vi "HFRR ADV v02.vi"() -> ()   [LabVIEW 2023] (continued)
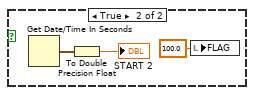
[diagram p4: hidden frame]
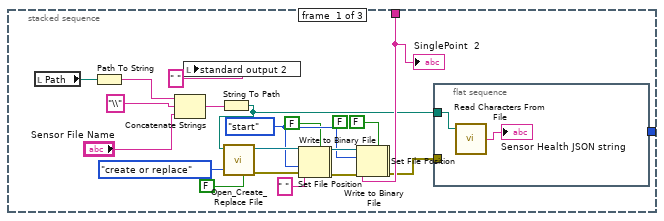
[diagram p9: hidden frame]
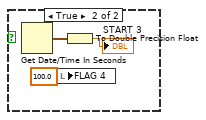
[diagram p13: hidden frame]
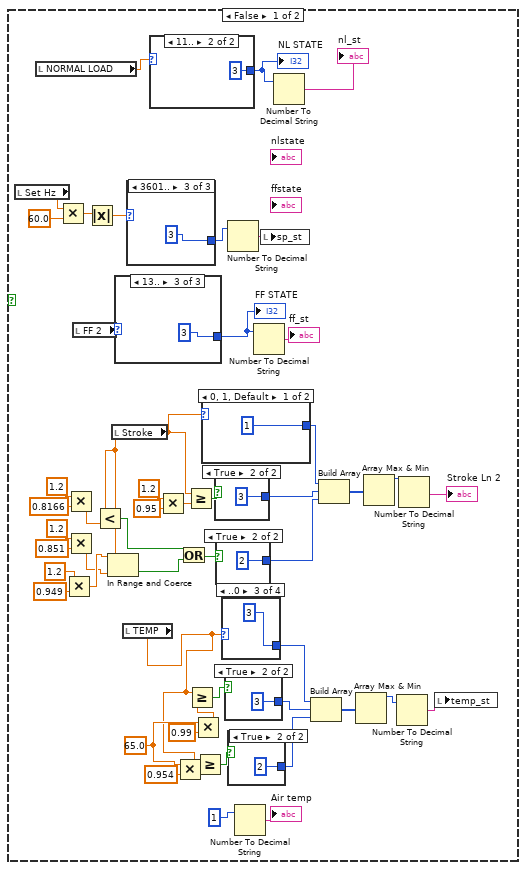
[diagram p15: hidden frame]
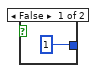
[diagram p16: hidden frame]
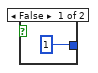
[diagram p17: hidden frame]
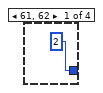
[diagram p18: hidden frame]
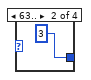
[diagram p19: hidden frame]
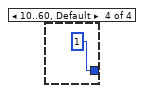
[diagram p20: hidden frame]
                n2644 = Multiply(x=1.2 ("y"), y=0.8166) -> (x*y=w3925:dbl)
                n2645 = Multiply(x=1.2 ("y"), y=0.851) -> (x*y=w3920:dbl)
                n2646 = local read "FF 2"() -> (w3944:dbl)
                n2647 = Absolute Value(x=w3952) -> (abs(x)=w3950:dbl)
                n2648 = local read "Stroke"() -> (w3919:dbl)
                n2649 = Less?(x=w3919, y=w3925) -> (x < y?=w3922:bool)
                n2650 = In Range and Coerce(upper limit=w3921, x=w3919, lower limit=w3920) -> (In Range?=w3923:bool)  [unwired: 1 out]
                n2651 = case shown="13.." w3944 {
                  tunnel: [1 2 3] -> w3942
                  frame 0..10, Default {
                    # "Normal"
                  }
                  frame 11, 12 {
                  }
                  frame 13.. {
                  }
                }
                "FF STATE" <- w3942
                n2652 = local read "TEMP"() -> (w3905:dbl)
                n2653 = case shown="3601.." w3950 {
                  tunnel: [1 2 3] -> w3948
                  frame 0..3000, Default {
                    # "Normal"
                  }
                  frame 3001..3600 {
                  }
                  frame 3601.. {
                  }
                }
                n2654 = case shown="11.." w3946 {
                  tunnel: [1 3] -> w3947
                  frame 1..10, Default {
                  }
                  frame 11.. {
                  }
                }
                "NL STATE" <- w3947
                n2655 = Multiply(x=1.2 ("y"), y=0.95) -> (x*y=w3935:dbl)
                n2656 = Multiply(x=w3917, y=0.954) -> (x*y=w3909:dbl)
                n2657 = Or(x=w3922, y=w3923) -> (x .or. y?=w3924:bool)
                n2658 = Greater Or Equal?(x=w3919, y=w3935) -> (x >= y?=w3932:bool)
                n2659 = Multiply(x=w3917, y=0.99) -> (x*y=w3906:dbl)
                n2660 = Greater Or Equal?(x=w3905, y=w3906) -> (x >= y?=w3911:bool)
                n2661 = Greater Or Equal?(x=w3905, y=w3909) -> (x >= y?=w3908:bool)
                n2662 = case shown="0, 1, Default" w3919 {
                  tunnel: [1 3] -> w3936
                  frame 0, 1, Default {
                  }
                  frame 2.. {
                  }
                }
                n2663 = case shown="True" w3932 {
                  tunnel: [1 3] -> w3937
                  frame False {
                  }
                  frame True {
                  }
                }
                n2664 = case shown="True" w3924 {
                  tunnel: [1 2] -> w3938
                  frame False {
                  }
                  frame True {
                  }
                }
                n2665 = case shown="..0" w3905 {
                  tunnel: [2 3 3 1] -> w3912
                  frame 61, 62 {
                  }
                  frame 63.. {
                  }
                  frame ..0 {
                  }
                  frame 10..60, Default {
                  }
                }
                n2666 = case shown="True" w3911 {
                  tunnel: [1 3] -> w3913
                  frame False {
                  }
                  frame True {
                  }
                }
                n2667 = Number To Decimal String(number=w3948) -> (decimal integer string=w3949:string)  [unwired: 1 in]
                n2668 = case shown="True" w3908 {
                  tunnel: [1 2] -> w3914
                  frame False {
                  }
                  frame True {
                  }
                }
                n2669 = Number To Decimal String(number=1) -> (decimal integer string=→"Air temp":string)  [unwired: 1 in]
                n2670 = Number To Decimal String(number=w3942) -> (decimal integer string=→"ff_st":string)  [unwired: 1 in]
                n2671 = local write "sp_st"(w3949) -> ()
                n2672 = Number To Decimal String(number=w3947) -> (decimal integer string=→"nl_st":string)  [unwired: 1 in]
                n2673 = Build Array(w3912, w3913, w3914) -> (w3915:i32[])
                n2674 = Build Array(w3936, w3937, w3938) -> (w3939:i32[])
                n2675 = Array Max & Min(array=w3915) -> (max value=w3916:i32)  [unwired: 3 out]
                n2676 = Array Max & Min(array=w3939) -> (max value=w3940:i32)  [unwired: 3 out]
                n2677 = Number To Decimal String(number=w3916) -> (decimal integer string=w3904:string)  [unwired: 1 in]
                n2678 = Number To Decimal String(number=w3940) -> (decimal integer string=→"Stroke Ln 2":string)  [unwired: 1 in]
                n2679 = local write "temp_st"(w3904) -> ()
              }
              frame True {
                w4002 = 65.0 ("y")
                # "Healthy -1\nWarning -2\nError -3"
                n2680 = local read "TEMP"() -> (w4013:dbl)
                n2681 = local read "NORMAL LOAD"() -> (w4017:dbl)
                n2682 = local read "Set Hz"() -> (w4015:dbl)
                n2683 = Multiply(x=1.2 ("y"), y=0.949) -> (x*y=w3997:dbl)
                n2684 = Multiply(x=1.2 ("y"), y=0.8166) -> (x*y=w3993:dbl)
                n2685 = Multiply(x=1.2 ("y"), y=0.851) -> (x*y=w3998:dbl)
                n2686 = Multiply(x=w4002, y=0.954) -> (x*y=w4009:dbl)
                n2687 = Multiply(x=w4002, y=0.99) -> (x*y=w4012:dbl)
                n2688 = Greater Or Equal?(x=w4013, y=w4012) -> (x >= y?=w4007:bool)
                n2689 = Multiply(x=w4015, y=60.0) -> (x*y=w4021:dbl)
                n2690 = Greater Or Equal?(x=w4013, y=w4009) -> (x >= y?=w4010:bool)
                n2691 = local read "FF 2"() -> (w4016:dbl)
                n2692 = local read "Stroke"() -> (w3999:dbl)
                n2693 = Less?(x=w3999, y=w3993) -> (x < y?=w3996:bool)
                n2694 = In Range and Coerce(upper limit=w3997, x=w3999, lower limit=w3998) -> (In Range?=w3995:bool)  [unwired: 1 out]
                n2695 = Absolute Value(x=w4021) -> (abs(x)=w4019:dbl)
                n2696 = case shown="63.." w4013 {
                  tunnel: [2 3 3 1] -> w4006
                  frame 61, 62 {
                  }
                  frame 63.. {
                  }
                  frame ..0 {
                  }
                  frame 10..60, Default {
                  }
                }
                n2697 = case shown="True" w4007 {
                  tunnel: [1 3] -> w4005
                  frame False {
                  }
                  frame True {
                  }
                }
                n2698 = case shown="True" w4010 {
                  tunnel: [1 2] -> w4004
                  frame False {
                  }
                  frame True {
                  }
                }
                n2699 = Multiply(x=1.2 ("y"), y=0.95) -> (x*y=w3983:dbl)
                n2700 = case shown="1..10, Default" w4017 {
                  tunnel: [1 3] -> w4024
                  frame 1..10, Default {
                  }
                  frame 11.. {
                  }
                }
                n2701 = case shown="0..10, Default" w4016 {
                  tunnel: [1 2 3] -> w4023
                  frame 0..10, Default {
                  }
                  frame 11, 12 {
                  }
                  frame 13.. {
                  }
                }
                n2702 = case shown="3601.." w4019 {
                  tunnel: [1 2 3] -> w4018
                  frame 0..3000, Default {
                    # "Normal"
                  }
                  frame 3001..3600 {
                  }
                  frame 3601.. {
                  }
                }
                n2703 = Or(x=w3996, y=w3995) -> (x .or. y?=w3994:bool)
                n2704 = Greater Or Equal?(x=w3999, y=w3983) -> (x >= y?=w3986:bool)
                n2705 = case shown="0, 1, Default" w3999 {
                  tunnel: [1 3] -> w3982
                  frame 0, 1, Default {
                  }
                  frame 2.. {
                  }
                }
                n2706 = case shown="True" w3986 {
                  tunnel: [1 3] -> w3981
                  frame False {
                  }
                  frame True {
                  }
                }
                n2707 = case shown="True" w3994 {
                  tunnel: [1 2] -> w3980
                  frame False {
                  }
                  frame True {
                  }
                }
                n2708 = Build Array(w4006, w4005, w4004) -> (w4003:i32[])
                n2709 = Number To Decimal String(number=w4018) -> (decimal integer string=→"sp_st":string)  [unwired: 1 in]
                n2710 = Array Max & Min(array=w4003) -> (max value=w4000:i32)  [unwired: 3 out]
                "TEMP STATE" <- w4000
                n2711 = Number To Decimal String(number=w4024) -> (decimal integer string=w4027:string)  [unwired: 1 in]
                n2712 = Number To Decimal String(number=w4023) -> (decimal integer string=w4025:string)  [unwired: 1 in]
                n2713 = Number To Decimal String(number=w4000) -> (decimal integer string=→"temp_st":string)  [unwired: 1 in]
                n2714 = Build Array(w3982, w3981, w3980) -> (w3979:i32[])
                n2715 = local write "nl_st"(w4027) -> ()
                n2716 = local write "ff_st"(w4025) -> ()
                n2717 = Number To Decimal String(number=1) -> (decimal integer string=w4022:string)  [unwired: 1 in]
                n2718 = Array Max & Min(array=w3979) -> (max value=w3978:i32)  [unwired: 3 out]
                n2719 = local write "Air temp"(w4022) -> ()
                n2720 = Number To Decimal String(number=w3978) -> (decimal integer string=w3977:string)  [unwired: 1 in]
                n2721 = local write "Stroke Ln 2"(w3977) -> ()
              }
            }
            n2722 = local read "Stroke Ln 2"() -> (w3889:string)
            n2723 = local read "nl_st"() -> (w3895:string)
            n2724 = local read "ff_st"() -> (w3892:string)
            n2725 = local read "sp_st"() -> (w3893:string)
            n2726 = local read "temp_st"() -> (w3894:string)
            n2727 = local read "Air temp"() -> (w3888:string)
            n2728 = Replace Array Subset(array="in", new element #1=w3895, index #1=1 ("index"), new element #2=w3892, index #2=2 ("index"), new element #3=w3894, index #3=3 ("index"), new element #4=w3893, index #4=4 ("index"), new element #5=w3889, index #5=5 ("index"), new element #6=w3888, index #6=6 ("index"), new element #7="Sensor State" ("new element/subarray"), index #7=0 ("index")) -> (→"out":string[])
          }
        }
        n2729 = Wait (ms)(milliseconds to wait=u32 10) -> ()  [unwired: 1 out]
        n2730 = local read "EXIT"() -> (w3884:bool)
      }
      n2731 = while {
        stop <- w3858 stop-if-true
        n2732 = local read "run replace"() -> (w3860:bool)
        n2733 = Wait (ms)(milliseconds to wait=u32 100) -> ()  [unwired: 1 out]
        n2734 = Equal?(x="FLAG 2", y=0.0) -> (x = y?=w3861:bool)
        n2735 = case shown="True" w3861 {
          frame False {
          }
          frame True {
            n2736 = local write "FLAG 2"(100.0 ("FLAG 2")) -> ()
            n2737 = call <vilib>:"Read Characters From File.vi"("file path (dialog if empty)"=path "C:/LAB-IQ-NXT/WO 2449 TT.sig", "convert eol? (no:F)"=FALSE ("append to file? (new file:F)")) -> ("character string"=w3864:string)  [unwired: 4 in, 3 out]
            n2738 = call <vilib>:"Read Characters From File.vi"("file path (dialog if empty)"=path "C:/LAB-IQ-NXT/WO 2449 TRH.sig", "convert eol? (no:F)"=FALSE ("append to file? (new file:F)")) -> ("character string"=w3865:string)  [unwired: 4 in, 3 out]
            n2739 = Decimal String To Number(string=w3864) -> (number=w3866:i32)  [unwired: 2 in, 1 out]
            n2740 = local write "Total No. of Tests"(w3866) -> ()
            n2741 = Decimal String To Number(string=w3865) -> (number=w3869:i32)  [unwired: 2 in, 1 out]
            n2742 = local write "SEN.RUN HRS"(w3869) -> ()
          }
        }
        n2743 = case shown="True" w3860 {
          frame False {
          }
          frame True {
            n2744 = Equal?(x="FLAG 4", y=0.0) -> (x = y?=w3873:bool)
            n2745 = case shown="False" w3873 {
              frame False {
                n2746 = Get Date/Time In Seconds() -> (seconds since 1Jan1904=w3879:timestamp)
                n2747 = local read "START 3"() -> (w3877:dbl)
                n2748 = To Double Precision Float(number=w3879) -> (double precision float=w3878:dbl)
                n2749 = Subtract(x=w3878, y=w3877) -> (x-y=→"SENSOR TIME":dbl)
              }
              frame True {
                n2750 = Get Date/Time In Seconds() -> (seconds since 1Jan1904=w3881:timestamp)
                n2751 = local write "FLAG 4"(100.0 ("FLAG")) -> ()
                n2752 = To Double Precision Float(number=w3881) -> (double precision float=→"START 3":dbl)
              }
            }
          }
        }
        n2753 = local read "EXIT"() -> (w3858:bool)
      }
      n2754 = while {
        shift-right: [w3656] -> _
        shift-left: _ -> [w3657]
        tunnel: [w3651] -> _
        i -> [w3651]
        stop <- w3650 stop-if-true
        n2755 = Wait (ms)(milliseconds to wait=u32 50 ("Refresh Rate (ms)")) -> ()  [unwired: 1 out]
        n2756 = local read "Json End Flg"() -> (w3652:bool)
        n2757 = Not(x="Upld AR 2") -> ()  [unwired: 1 out]
        n2758 = local read "Upld AR 2"() -> (w3653:bool)
        n2759 = call "Elapsed Time9"("Time Target (s)"="Sen.Upload Rate (s)", "Reset"=FALSE, "Auto Reset"=TRUE) -> ("Time has Elapsed"=w3663:bool)  [unwired: 9 in, 7 out]
        n2760 = Or(x=w3663, y=w3652) -> (x .or. y?=w3659:bool)
        n2761 = case shown="True" w3659 {
          frame False {
          }
          frame True {
            w3757 = "\"SensorName\":\"" ("string")
            w3727 = " \"},{"
            w3752 = "\",\"SensorState\":\""
            w3754 = "\",\"SensorModelNumber\":\"" ("string")
            w3753 = "\",\"SensorRuntimeHours\":\"" ("string")
            n2762 = local read "model num"() -> (w3751:string[])
            n2763 = local read "Sensor name"() -> (w3770:string[])
            n2764 = local read "run"() -> (w3741:string[])
            n2765 = local read "SENSOR TIME"() -> (w3696:dbl)
            n2766 = local read "out"() -> (w3689:string[])
            n2767 = local read "Total No. of Tests"() -> (w3694:dbl)
            n2768 = Select(t=60.0, s="Run test 3", f=3600.0) -> (s? t:f=w3705:dbl)
            n2769 = Index Array(array=w3751, index #1=1 ("index")) -> (element #1=w3750:string, element #2=w3749:string, element #3=w3748:string, element #4=w3747:string, element #5=w3746:string, element #6=w3745:string)  [unwired: 5 in]
            n2770 = Index Array(array=w3741, index #1=1 ("index")) -> (element #1=w3740:string, element #2=w3739:string, element #3=w3738:string, element #4=w3737:string, element #5=w3736:string, element #6=w3735:string)  [unwired: 5 in]
            n2771 = Index Array(array=w3770, index #1=1 ("index")) -> (element #1=w3769:string, element #2=w3768:string, element #3=w3767:string, element #4=w3766:string, element #5=w3756:string, element #6=w3755:string)  [unwired: 5 in]
            n2772 = Index Array(array=w3689, index #1=1 ("index")) -> (element #1=w3722:string, element #2=w3721:string, element #3=w3720:string, element #4=w3719:string, element #5=w3718:string, element #6=w3717:string)  [unwired: 5 in]
            n2773 = local read "SEN.RUN HRS"() -> (w3692:dbl)
            n2774 = Divide(x=w3696, y=w3705) -> (x/y=w3704:dbl)
            n2775 = Increment(x=w3704) -> (x+1=w3699:dbl)
            n2776 = Number To Decimal String(number=w3699) -> (decimal integer string=→"run hrs":string)  [unwired: 1 in]
            n2777 = Divide(x=w3692, y=3600.0 ("f")) -> (x/y=w3687:dbl)
            n2778 = Round To Nearest(number=w3687) -> (nearest integer value=w3685:dbl)
            n2779 = Number To Decimal String(number=w3685) -> (decimal integer string=w3686:string)  [unwired: 1 in]
            n2780 = Number To Decimal String(number=w3694) -> (decimal integer string=w3695:string)  [unwired: 1 in]
            n2781 = local read "Model No"() -> (w3700:string)
            n2782 = local read "UUID"() -> (w3796:string)
            n2783 = local read "Serial No"() -> (w3800:string)
            n2784 = local read "Secret Key"() -> (w3801:string)
            n2785 = Concatenate Strings("\",\"MachineSerialNumber\":\"" ("string"), w3800) -> (w3804:string)
            n2786 = Concatenate Strings("\",\"ModelNumber\":\"" ("string"), w3700) -> (w3701:string)
            n2787 = Concatenate Strings("\",\"MachineRuntimeHours\":\"" ("string"), w3686) -> (w3805:string)
            n2788 = Concatenate Strings("\",\"MachineRuntimeCycles\":\"", w3695) -> (w3798:string)
            n2789 = Concatenate Strings(w3754, w3750) -> (w3784:string)
            n2790 = Concatenate Strings(w3753, w3740) -> (w3785:string)
            n2791 = Concatenate Strings(w3752, w3722) -> (w3783:string)
            n2792 = Concatenate Strings(w3804, w3701, w3805, w3798) -> (w3807:string)
            n2793 = Concatenate Strings(w3754, w3749) -> (w3781:string)
            n2794 = Concatenate Strings(w3753, w3739) -> (w3780:string)
            n2795 = Concatenate Strings(w3752, w3721) -> (w3782:string)
            n2796 = Concatenate Strings(w3754, w3748) -> (w3776:string)
            n2797 = Concatenate Strings(w3753, w3738) -> (w3777:string)
            n2798 = Concatenate Strings(w3752, w3720) -> (w3775:string)
            n2799 = Concatenate Strings(w3754, w3747) -> (w3773:string)
            n2800 = Concatenate Strings(w3753, w3737) -> (w3772:string)
            n2801 = Concatenate Strings(w3752, w3719) -> (w3774:string)
            n2802 = Concatenate Strings(w3784, w3785, w3783) -> (w3786:string)
            n2803 = Concatenate Strings(w3754, w3746) -> (w3763:string)
            n2804 = Concatenate Strings(w3753, w3736) -> (w3764:string)
            n2805 = Concatenate Strings(w3754, w3745) -> (w3760:string)
            n2806 = Concatenate Strings(w3753, w3735) -> (w3759:string)
            n2807 = Concatenate Strings(w3752, w3718) -> (w3762:string)
            n2808 = Concatenate Strings(w3752, w3717) -> (w3761:string)
            n2809 = Concatenate Strings("{\"SecretKey\":\"", w3801, w3807, "\",\"UUID\" : \"", w3796, "\",\"SensorInformation\":", "[{" ("string")) -> (w3734:string)
            n2810 = Concatenate Strings(w3781, w3780, w3782) -> (w3779:string)
            n2811 = Concatenate Strings(w3776, w3777, w3775) -> (w3778:string)
            n2812 = Concatenate Strings(w3773, w3772, w3774) -> (w3771:string)
            n2813 = Concatenate Strings(w3763, w3764, w3762) -> (w3765:string)
            n2814 = Concatenate Strings(w3760, w3759, w3761) -> (w3758:string)
            n2815 = Concatenate Strings(w3757, w3769, w3786, w3727) -> (w3733:string)
            n2816 = Concatenate Strings(w3757, w3768, w3779, w3727) -> (w3732:string)
            n2817 = Concatenate Strings(w3757, w3767, w3778, w3727) -> (w3731:string)
            n2818 = Concatenate Strings(w3757, w3766, w3771, w3727) -> (w3730:string)
            n2819 = Concatenate Strings(w3757, w3756, w3765, w3727) -> (w3729:string)
            n2820 = Concatenate Strings(w3757, w3755, w3758, "\"}" ("string")) -> (w3728:string)
            n2821 = Concatenate Strings(w3734, w3733, w3732, w3731, w3730, w3729, w3728, "]}" ("string")) -> (w3725:string)
            n2822 = local read "SEN.RUN HRS"() -> (w3691:dbl)
            n2823 = case shown="True" "Case Constant\n(See Context Help) 3" {
              frame False {
              }
              frame True {
                n2824 = local read "state"() -> (w3811:string[])
                n2825 = Delete From Array(array=w3811, index=0) -> (array with subset deleted=w3809:string[])  [unwired: 1 in, 1 out]
                n2826 = for {
                  N: 6 -> [_]
                  tunnel: w3809 -> [w3822] mode=indexing
                  tunnel: [w3821] -> w3808 mode=indexing
                  n2827 = Equal?(x=w3822, y="Warning") -> (x = y?=w3818:bool)
                  n2828 = Equal?(x=w3822, y="Healthy") -> (x = y?=w3815:bool)
                  n2829 = Select(t="2" ("y"), s=w3818, f="3" ("y")) -> (s? t:f=w3813:string)
                  n2830 = Select(t="1" ("y"), s=w3815, f=w3813) -> (s? t:f=w3821:string)
                }
                "state1" <- w3808
              }
            }
            n2831 = stacked-sequence {
              tunnel: w3725 -> [w3833 _ _]
              tunnel: [_ _ w3849] -> _
              frame #0 {
                (unwired) FALSE ("convert eol (F)")
                w3835 = enum16{"start", "end", "current"}."start" ("pos mode (0:2)")
                n2832 = local read "Path"() -> (w3829:path)
                n2833 = Path To String(path=w3829) -> (string=w3841:string)
                n2834 = Concatenate Strings(w3841, "\\", "Sensor File Name") -> (w3842:string)
                n2835 = local write "standard output 2"(" ") -> ()
                n2836 = String To Path(string=w3842) -> (path=w3832:path)
                n2837 = call <vilib>:"Open_Create_Replace File.vi"("advisory dialog? (display:T)"=FALSE, "function (open:0)"=T16."create or replace", "file path"=w3832) -> ("error out"=w3845:errorcluster, "refnum"=w3844:refnum<file>)  [unwired: 5 in, 2 out]
                n2838 = Set File Position(refnum=w3844, from (0:start)=w3835, error in=w3845) -> (refnum out=w3825:refnum<file>, error out=w3824:errorcluster)  [unwired: 1 in]
                n2839 = Write to Binary File(file (use dialog)=w3825, data=" ", error in=w3824, 5:FALSE ("prepend array or string size? (T)")) -> (refnum out=w3836:refnum<file>, error out=w3837:errorcluster)  [unwired: 2 in, 1 out]
                n2840 = Set File Position(offset (in bytes) (0)=w3835, refnum=w3836, error in=w3837) -> (refnum out=w3828:refnum<file>, error out=w3827:errorcluster)  [unwired: 1 in]
                n2841 = Write to Binary File(file (use dialog)=w3828, data=w3833, error in=w3827, 5:FALSE ("prepend array or string size? (T)")) -> (error out=w3831:errorcluster)  [unwired: 2 in, 2 out]
                n2842 = flat-sequence {
                  tunnel: w3832 -> [w3847]
                  tunnel: w3831 -> [_]
                  frame #0 {
                    n2843 = call <vilib>:"Read Characters From File.vi"("file path (dialog if empty)"=w3847) -> ("character string"=→"Sensor Health JSON string":string)  [unwired: 5 in, 3 out]
                  }
                }
                "SinglePoint  2" <- w3833
              }
              frame #1 {
              }
              frame #2 {
                (unwired) "\"Stored\": true" ("string")
                n2844 = call <vilib>:"System Exec.vi"("run minimized? (F)"=TRUE, "wait until completion? (T)"=TRUE, "working directory"=path "C:/LAB-IQ-NXT", "command line"="C:\\LAB-IQ-NXT\\JPostH.bat") -> ("standard error"=→"Respose From Server 2":string, "standard output"=w3852:string)  [unwired: 4 in, 2 out]
                "standard output 2" <- w3852
                n2845 = Match Pattern(string=w3852, regular expression="JSONH Check String") -> (match substring=w3850:string, offset past match=w3849:i32)  [unwired: 1 in, 2 out]
                n2846 = Equal?(x=w3850, y="JSONH Check String") -> (x = y?=→"Upload \nConfirmed 2":bool)
              }
            }
            n2847 = Divide(x=w3691, y=3600.0 ("f")) -> (x/y=w3684:dbl)
            n2848 = local read "run time"() -> (w3742:string[])
            n2849 = Round To Nearest(number=w3684) -> (nearest integer value=w3683:dbl)
            n2850 = Number To Decimal String(number=w3683) -> (decimal integer string=w3682:string)  [unwired: 1 in]
            n2851 = Index Array(array="Sensor Information", index (col) #1=0 ("disabled index (col)"), index (col) #2=1 ("index (col)"), index (col) #3=2 ("index (col)"), index (col) #4=3 ("index (col)")) -> (element #1=→"Sensor name":string[], element #2=→"model num":string[], element #3=→"run time":string[], element #4=→"state":string[])  [unwired: 4 in]
            n2852 = Insert Into Array(array=w3742, index=1, new element #1=w3682, new element #2=w3682, new element #3=w3682, new element #4=w3682, new element #5=w3682, new element #6=w3682) -> (w3707:string[])
            "run" <- w3707
            n2853 = local read "out"() -> (w3688:string[])
            n2854 = local read "Sensor Information"() -> (w3709:string[][])
            n2855 = Replace Array Subset(array=w3709, new element #1=w3707, index (col) #1=2 ("disabled index (col)"), new element #2=w3688, index (col) #2=3 ("index (col)")) -> (w3708:string[][])  [unwired: 2 in]
            n2856 = local write "Sensor Information"(w3708) -> ()
          }
        }
        n2857 = case shown="True" w3653 {
          frame False {
          }
          frame True {
            n2858 = Equal?(x="FLAG", y=0.0) -> (x = y?=w3664:bool)
            n2859 = case shown="False" w3664 {
              frame False {
                n2860 = Get Date/Time In Seconds() -> (seconds since 1Jan1904=w3670:timestamp)
                n2861 = local read "START 2"() -> (w3668:dbl)
                n2862 = To Double Precision Float(number=w3670) -> (double precision float=w3669:dbl)
                n2863 = Subtract(x=w3669, y=w3668) -> (x-y=→"SENSOR TIME  2":dbl)
              }
              frame True {
                n2864 = Get Date/Time In Seconds() -> (seconds since 1Jan1904=w3672:timestamp)
                n2865 = To Double Precision Float(number=w3672) -> (double precision float=→"START 2":dbl)
                n2866 = local write "FLAG"(100.0 ("FLAG")) -> ()
              }
            }
          }
        }
        n2867 = case shown="True" "Case Constant\n(See Context Help) 2" {
          tunnel: w3657 -> [w3674 w3676]
          tunnel: [w3674 w3675] -> w3656
          frame False {
          }
          frame True {
            n2868 = local read "Json St Flg"() -> (w3677:bool)
            n2869 = case shown="True" w3677 {
              tunnel: w3676 -> [w3678 w3680]
              tunnel: [w3678 w3679] -> w3675
              frame False {
              }
              frame True {
                n2870 = Increment(x=w3680) -> (x+1=w3679:dbl)
                "T cycle" <- w3679
                n2871 = local write "Json St Flg"(FALSE ("Json St Flg")) -> ()
              }
            }
          }
        }
        n2872 = local read "EXIT"() -> (w3650:bool)
      }
    }
  }
  n2873 = stacked-sequence {
    tunnel: [w4051] -> w17
    frame #0 {
      w4051 = FALSE ("Upload \nConfirmed")
      n2874 = local write "Upload \nConfirmed"(w4051) -> ()
      n2875 = local write "St Str"("") -> ()
    }
  }
  n2876 = case shown="True" "Case Constant\n(See Context Help) 4" {
    tunnel: w17 -> [_ w4052]
    frame False {
    }
    frame True {
      n2877 = while {
        tunnel: [w4058] -> _
        tunnel: w4052 -> [_]
        i -> [w4058]
        stop <- w4055 stop-if-true
        n2878 = local read "Json End Flg"() -> (w4057:bool)
        n2879 = Wait (ms)(milliseconds to wait=u32 20 ("Refresh Rate (ms)")) -> ()  [unwired: 1 out]
        n2880 = local read "refresh flag"() -> (w4053:bool)
        n2881 = local read "RUN"() -> (w4054:bool)
        n2882 = And(x=w4054, y=w4053) -> (x .and. y?=w4056:bool)
        n2883 = Or(x=w4056, y=w4057) -> (x .or. y?=w4059:bool)
        "AR Led" <- w4059
        n2884 = case shown="True" w4059 {
          frame False {
          }
          frame True {
            w4076 = "\",\""
            n2885 = local read "UUID"() -> (w4074:string)
            n2886 = local write "refresh flag"(FALSE ("refresh flag")) -> ()
            n2887 = local read "time"() -> (w4063:dbl)
            n2888 = Multiply(x=w4063, y=60.0) -> (x*y=w4062:dbl)
            n2889 = Concatenate Strings("UUID\" : \"", w4074, "\"}") -> (w4077:string)
            n2890 = Number To Fractional String(number=w4062, width (-)=i16 10, precision (6)=i16 4) -> (F-format string=w4091:string)  [unwired: 1 in]
            n2891 = Concatenate Strings("{", "\"Time\":\"", w4091, w4076) -> (w4086:string)
            n2892 = stacked-sequence {
              tunnel: w4076 -> [w4139 w4147 w4154 w4162 w4170 w4179 w4186]
              tunnel: [w4140 _ _ _ _ _ _] -> w4090
              tunnel: [_ w4148 _ _ _ _ _] -> w4089
              tunnel: [_ _ w4155 _ _ _ _] -> w4088
              tunnel: [_ _ _ w4164 _ _ _] -> w4087
              tunnel: w4077 -> [_ _ _ _ _ _ w4197]
              tunnel: [_ _ _ _ _ _ w4196] -> w4073
              tunnel: [_ _ _ _ _ w4176 _] -> w4072
              tunnel: [_ _ _ _ w4169 _ _] -> w4071
              frame #0 {
                n2893 = local read "NORMAL LOAD"() -> (w4138:dbl)
                n2894 = Number To Fractional String(number=w4138, width (-)=i16 10, precision (6)=i16 4) -> (F-format string=w4141:string)  [unwired: 1 in]
                n2895 = Concatenate Strings("NormalLoad\":\"", w4141, w4139) -> (w4140:string)
              }
              frame #1 {
                n2896 = local read "Temp"() -> (w4146:dbl)
                n2897 = Number To Fractional String(number=w4146, width (-)=i16 10, precision (6)=i16 4) -> (F-format string=w4149:string)  [unwired: 1 in]
                n2898 = Concatenate Strings("Temperature\":\"", w4149, w4147) -> (w4148:string)
              }
              frame #2 {
                n2899 = local read "cof"() -> (w4152:dbl)
                n2900 = Number To Fractional String(number=w4152, width (-)=i16 10, precision (6)=i16 4) -> (F-format string=w4156:string)  [unwired: 1 in]
                n2901 = Concatenate Strings("FrictionalForce\":\"", w4156, w4154) -> (w4155:string)
              }
              frame #3 {
                n2902 = local read "Set Hz"() -> (w4160:dbl)
                n2903 = Multiply(x=w4160, y=60.0) -> (x*y=w4159:dbl)
                n2904 = Number To Fractional String(number=w4159, width (-)=i16 10, precision (6)=i16 4) -> (F-format string=w4165:string)  [unwired: 1 in]
                n2905 = Concatenate Strings("Speed\":\"", w4165, w4162) -> (w4164:string)
              }
              frame #4 {
                n2906 = local read "Stroke Ln"() -> (w4168:dbl)
                n2907 = Number To Fractional String(number=w4168, width (-)=i16 10, precision (6)=i16 4) -> (F-format string=w4172:string)  [unwired: 1 in]
                n2908 = Concatenate Strings("LinearDeformation\":\"", w4172, w4170) -> (w4169:string)
              }
              frame #5 {
                n2909 = local read "AIR TEMP"() -> (w4175:dbl)
                n2910 = local read "Json St Flg"() -> (w4177:bool)
                n2911 = local read "Json End Flg"() -> (w4178:bool)
                n2912 = Number To Fractional String(number=w4175, width (-)=i16 10, precision (6)=i16 4) -> (F-format string=w4181:string)  [unwired: 1 in]
                n2913 = Concatenate Strings("Vibration\":\"", w4181, w4179) -> (w4176:string)
                n2914 = And(x=w4177, y=w4178) -> ()  [unwired: 1 out]
              }
              frame #6 {
                n2915 = local read "Json End Flg"() -> (w4185:bool)
                n2916 = Get Date/Time In Seconds() -> (seconds since 1Jan1904=w4193:timestamp)
                n2917 = local read "Json St Flg"() -> (w4184:bool)
                n2918 = To Double Precision Float(number=w4193) -> (double precision float=w4192:dbl)
                n2919 = Subtract(x=w4192, y=2082844800.0) -> (x-y=w4190:dbl)
                n2920 = Number To Fractional String(number=w4190, width (-)=i16 12, precision (6)=i16 0) -> (F-format string=w4187:string)  [unwired: 1 in]
                n2921 = case shown="True" w4185 {
                  tunnel: ["" w4200] -> w4194
                  tunnel: w4187 -> [_ w4201]
                  tunnel: w4186 -> [_ w4199]
                  frame False {
                  }
                  frame True {
                    n2922 = local write "Json End Flg"(FALSE ("Json St Flg")) -> ()
                    n2923 = Concatenate Strings("End\": \"", w4201, w4199) -> (w4200:string)
                  }
                }
                n2924 = case shown="True" w4184 {
                  tunnel: [w4204 w4207] -> w4195
                  tunnel: w4187 -> [_ w4208]
                  tunnel: w4186 -> [_ w4205]
                  frame False {
                    n2925 = local read "St Str"() -> (w4204:string)
                  }
                  frame True {
                    n2926 = Concatenate Strings("Start\":\"", w4208, w4205) -> (w4207:string)
                    "St Str" <- w4207
                    n2927 = local write "Json St Flg"(FALSE ("Json St Flg")) -> ()
                  }
                }
                n2928 = Concatenate Strings(w4195, w4194, w4197) -> (w4196:string)
              }
            }
            n2929 = local read "FILE"() -> (w4065:string)
            n2930 = Concatenate Strings("\",\"OperatorID\":\"" ("string"), "Operator ID") -> (w4068:string)
            n2931 = Concatenate Strings("\",\"DatasetTitle\":\"" ("string"), w4065) -> (w4067:string)
            n2932 = Concatenate Strings("\",\"SerialNumber\":\"" ("string"), "Serial No") -> (w4097:string)
            n2933 = Concatenate Strings("\",\"ModelNumber\":\"" ("string"), "Model No") -> (w4096:string)
            n2934 = Concatenate Strings(w4097, w4096) -> (w4079:string)
            n2935 = Concatenate Strings("{\"SecretKey\":\"", "Secret Key", w4079, w4068, w4067, "\",\"Samples\":[") -> (w4084:string)
            n2936 = Concatenate Strings(w4086, w4090, w4089, w4088, w4087, w4071, w4072, w4073) -> (w4085:string)
            n2937 = Concatenate Strings(w4084, w4085, "]}") -> (w4083:string)
            n2938 = stacked-sequence {
              tunnel: w4083 -> [w4112 _ _]
              tunnel: [_ _ w4129] -> _
              frame #0 {
                (unwired) FALSE ("convert eol (F)")
                w4114 = enum16{"start", "end", "current"}."start" ("pos mode (0:2)")
                n2939 = Path To String(path="Path") -> (string=w4120:string)
                n2940 = Concatenate Strings(w4120, "\\", "Data File Name") -> (w4122:string)
                n2941 = local write "standard output"(" ") -> ()
                n2942 = String To Path(string=w4122) -> (path=w4111:path)
                n2943 = call <vilib>:"Open_Create_Replace File.vi"("advisory dialog? (display:T)"=FALSE, "function (open:0)"=T16."create or replace", "file path"=w4111) -> ("error out"=w4125:errorcluster, "refnum"=w4124:refnum<file>)  [unwired: 5 in, 2 out]
                n2944 = Set File Position(refnum=w4124, from (0:start)=w4114, error in=w4125) -> (refnum out=w4105:refnum<file>, error out=w4104:errorcluster)  [unwired: 1 in]
                n2945 = Write to Binary File(file (use dialog)=w4105, data=" ", error in=w4104, 5:FALSE ("prepend array or string size? (T)")) -> (refnum out=w4115:refnum<file>, error out=w4116:errorcluster)  [unwired: 2 in, 1 out]
                n2946 = Set File Position(offset (in bytes) (0)=w4114, refnum=w4115, error in=w4116) -> (refnum out=w4108:refnum<file>, error out=w4107:errorcluster)  [unwired: 1 in]
                n2947 = Write to Binary File(file (use dialog)=w4108, data=w4112, error in=w4107, 5:FALSE ("prepend array or string size? (T)")) -> (error out=w4110:errorcluster)  [unwired: 2 in, 2 out]
                n2948 = flat-sequence {
                  tunnel: w4111 -> [w4127]
                  tunnel: w4110 -> [_]
                  frame #0 {
                    n2949 = call <vilib>:"Read Characters From File.vi"("file path (dialog if empty)"=w4127) -> ("character string"=→"JSON string":string)  [unwired: 5 in, 3 out]
                  }
                }
                "SinglePoint" <- w4112
              }
              frame #1 {
              }
              frame #2 {
                (unwired) "\"Stored\": true" ("string")
                n2950 = call <vilib>:"System Exec.vi"("run minimized? (F)"=TRUE, "wait until completion? (T)"=TRUE, "working directory"=path "C:/LAB-IQ-NXT", "command line"="C:\\LAB-IQ-NXT\\JPost.bat") -> ("standard error"=→"Respose From Server":string, "standard output"=w4132:string)  [unwired: 4 in, 2 out]
                "standard output" <- w4132
                n2951 = Match Pattern(string=w4132, regular expression="JSON Check String") -> (match substring=w4130:string, offset past match=w4129:i32)  [unwired: 1 in, 2 out]
                n2952 = Equal?(x=w4130, y="JSON Check String") -> (x = y?=→"Upload \nConfirmed":bool)
              }
            }
          }
        }
        n2953 = local read "EXIT"() -> (w4055:bool)
      }
    }
  }
  n2954 = case shown="True" "Case Constant\n(See Context Help) 8" {
    tunnel: w16 -> [_ w4210]
    frame False {
    }
    frame True {
      n2955 = while {
        shift-right: [w4223] -> w4212
        shift-left: _ -> [w4224]
        shift-right: [w4221] -> w4213
        shift-left: errorcluster {"status"=TRUE, "code"=0, "source"="Init"} ("error out") -> [w4222]
        shift-right: [w4219] -> _
        shift-left: "" -> [w4220]
        tunnel: [w4217] -> _
        tunnel: w4210 -> [_]
        i -> [w4217]
        stop <- w4216 stop-if-true
        n2956 = flat-sequence {
          tunnel: [w4225] -> w4218
          frame #0 {
            n2957 = Wait (ms)(milliseconds to wait=10.0 ("Delay")) -> (millisecond timer value=w4225:u32)
          }
        }
        n2958 = case shown="No Error" w4222 {
          selector: w4222 -> [w4258 w4380]
          tunnel: [w4240 w4382] -> w4223
          tunnel: [w4239 w4381] -> w4221
          tunnel: w4224 -> [w4259 w4374]
          tunnel: w4220 -> [w4238 w4373]
          tunnel: [w4237 w4373] -> w4219
          tunnel: w4218 -> [_ _]
          frame No Error {
            n2959 = Concatenate Strings("COMMAND", "\r", "\n") -> (w4249:string)
            n2960 = case shown="True" "Measure" {
              tunnel: w4259 -> [w4285 w4292]
              tunnel: w4258 -> [w4284 w4291]
              tunnel: [w4285 w4290] -> w4257
              tunnel: [w4284 w4289] -> w4236
              tunnel: w4249 -> [_ w4288]
              frame False {
              }
              frame True {
                n2961 = VISA Write(VISA resource name=w4292, write buffer=w4288, error in (no error)=w4291) -> (VISA resource name out=w4290:refnum<visa-resource-name>, error out=w4289:errorcluster)  [unwired: 1 out]
                n2962 = local write "Read String"("") -> ()
                n2963 = local write "Measure"(FALSE) -> ()
              }
            }
            n2964 = property class="Instr"(reference=w4257, error in=w4236) -> (reference out=w4256:refnum<visa-resource-name>, error out=w4255:errorcluster, "Serial Settings:Number of Bytes at Serial Port"=w4254:u32)
            n2965 = Greater?(x=w4254, y=u32 100) -> (0:w4252:bool)
            n2966 = case shown="True" w4252 {
              tunnel: w4256 -> [w4295 w4320]
              tunnel: w4255 -> [w4294 w4319]
              tunnel: w4254 -> [_ w4318]
              tunnel: [w4295 w4317] -> w4242
              tunnel: [w4294 w4316] -> w4241
              tunnel: w4238 -> [w4293 w4315]
              tunnel: [w4293 ""] -> w4237
              frame False {
              }
              frame True {
                w4305 = u32 6 ("y")
                # "Page 84 of \nmanual"
                n2967 = VISA Read(VISA resource name=w4320, byte count=w4318, error in (no error)=w4319) -> (VISA resource name out=w4317:refnum<visa-resource-name>, read buffer=w4313:string, error out=w4316:errorcluster)  [unwired: 1 out]
                n2968 = while {
                  tunnel: w4313 -> [w4369]
                  tunnel: [w4365] -> w4307 mode=indexing
                  tunnel: [w4359] -> w4311 mode=indexing
                  tunnel: [w4357] -> _
                  i -> [w4357]
                  stop <- w4362 stop-if-true
                  n2969 = String Subset(string=w4369, offset (0)=w4357) -> (substring=w4364:string)  [unwired: 1 in]
                  n2970 = String To Byte Array(string=w4364) -> (unsigned byte array=w4368:u8[])
                  n2971 = String Length(string=w4364) -> (length=w4363:i32)
                  n2972 = Index Array(array=w4368) -> (element=w4367:u8)  [unwired: 1 in]
                  n2973 = Equal To 0?(x=w4363) -> (x = 0?=w4362:bool)
                  n2974 = Number To Boolean Array(number=w4367) -> (Boolean array=w4361:bool[])
                  n2975 = Reverse 1D Array(array=w4361) -> (reversed array=w4360:bool[])
                  n2976 = And(x=w4361, y=bool[] [FALSE, FALSE, FALSE, FALSE, FALSE, FALSE, TRUE, TRUE] ("Boolean array")) -> (x .and. y?=w4365:bool[])
                  n2977 = And(x=w4360, y=bool[] [FALSE, FALSE, TRUE, TRUE, TRUE, TRUE, TRUE, TRUE] ("Boolean array")) -> (x .and. y?=w4359:bool[])
                }
                n2978 = Concatenate Strings(w4315, w4313) -> (→"Read String":string)
                n2979 = while {
                  tunnel: w4307 -> [w4356] mode=indexing
                  tunnel: [w4352] -> w4310
                  i -> [w4352]
                  stop <- w4353 stop-if-true
                  n2980 = Search 1D Array(1D array=w4356, element=TRUE) -> (index of element=w4354:i32)  [unwired: 1 in]
                  n2981 = Less Than 0?(x=w4354) -> (x < 0?=w4353:bool)
                }
                n2982 = Delete From Array(array=w4311, length=w4310, index (row)=0) -> (array with subset deleted=w4306:bool[][])  [unwired: 1 in, 1 out]
                n2983 = Array Size(array=w4306) -> (size(s)=w4308:i32[])
                n2984 = Index Array(array=w4308) -> (element=w4300:i32)  [unwired: 1 in]
                n2985 = Greater?(x=w4300, y=w4305) -> (0:w4303:bool)
                n2986 = Subtract(x=w4300, y=w4305) -> (x-y=w4304:u32)
                n2987 = Select(t=w4304, s=w4303, f=u32 0) -> (s? t:f=w4301:u32)
                n2988 = while {
                  tunnel: w4306 -> [w4339]
                  tunnel: [w4341] -> w4299 mode=indexing
                  tunnel: w4301 -> [w4323]
                  i -> [w4340]
                  stop <- w4338 stop-if-true
                  w4330 = 6 ("index")
                  w4329 = 2 ("length")
                  # "Page 65 of \nmanual"
                  n2989 = Multiply(x=u32 3 ("y"), y=w4340) -> (x*y=w4337:u32)
                  n2990 = Divide(x=u32 102 ("y"), y=u32 65520) -> (x/y=w4347:dbl)
                  n2991 = Greater Or Equal?(x=w4337, y=w4323) -> (x >= y?=w4338:bool)
                  n2992 = Index Array(array=w4339, index (row) #1=w4337) -> (element #1=w4335:bool[], element #2=w4334:bool[], element #3=w4333:bool[])  [unwired: 5 in]
                  n2993 = Reverse 1D Array(array=w4335) -> (reversed array=w4328:bool[])
                  n2994 = Reverse 1D Array(array=w4334) -> (reversed array=w4332:bool[])
                  n2995 = Reverse 1D Array(array=w4333) -> (reversed array=w4331:bool[])
                  n2996 = Delete From Array(array=w4328, length=w4329, index=w4330) -> (array with subset deleted=w4324:bool[])  [unwired: 1 out]
                  n2997 = Delete From Array(array=w4332, length=w4329, index=w4330) -> (array with subset deleted=w4325:bool[])  [unwired: 1 out]
                  n2998 = Delete From Array(array=w4331, length=w4329, index=w4330) -> (array with subset deleted=w4326:bool[])  [unwired: 1 out]
                  n2999 = Insert Into Array(array=bool[] [] ("Boolean array"), new element #1=w4324, new element #2=w4325, new element #3=w4326) -> (w4327:bool[])  [unwired: 1 in]
                  n3000 = Boolean Array To Number(Boolean array=w4327) -> (number=w4336:u32)
                  n3001 = Multiply(x=w4347, y=w4336) -> (x*y=w4346:dbl)
                  n3002 = Decrement(x=w4346) -> (x-1=w4345:dbl)
                  n3003 = Divide(x=w4345, y=u32 100) -> (x/y=w4343:dbl)
                  n3004 = Multiply(x=w4343, y=u32 10) -> (x*y=w4341:dbl)
                }
                n3005 = Delete From Array(array=w4299) -> (array with subset deleted=w4298:dbl[])  [unwired: 2 in, 1 out]
                "Waveform Graph 5" <- w4298
                "Waveform Chart 3" <- w4298
                n3006 = call-poly <vilib>:"Mean.vi"("X"=w4298) -> ("mean"=w4297:dbl)  [unwired: 1 out]
                "Measure_LDS" <- w4297
                n3007 = case shown="True" "Zero 4" {
                  tunnel: w4297 -> [_ w4322]
                  frame False {
                  }
                  frame True {
                    n3008 = local write "Zero 4"(FALSE ("Zero 4")) -> ()
                    "z_measure" <- w4322
                  }
                }
              }
            }
            n3009 = local read "Measure_LDS"() -> (w4232:dbl)
            n3010 = local read "Disp (mm)"() -> (w4231:dbl)
            n3011 = local read "Boolean 7"() -> (w4230:bool)
            n3012 = local read "Boolean 8"() -> (w4229:bool)
            n3013 = case shown="True" "Boolean 8" {
              tunnel: w4231 -> [_ w4262]
              tunnel: w4232 -> [_ w4261]
              frame False {
              }
              frame True {
                n3014 = local read "Captured Values 2"() -> (w4265:dbl[][])
                n3015 = Build Array(w4262, w4261) -> (w4260:dbl[])
                n3016 = Build Array (concatenate)(w4265, w4260) -> (w4263:dbl[][])
                n3017 = local write "Captured Values 2"(w4263) -> ()
                n3018 = local write "Boolean 8"(FALSE ("Boolean 8")) -> ()
              }
            }
            n3019 = call "Build XY Graph"("Enable"=w4229, "Reset"=w4230, "Y Input"=w4232, "X Input"=w4231) -> ("XY Graph"=→"?":cluster{"Y":dbl[], "Y":dbl[]}[])  [unwired: 6 in, 1 out]
            n3020 = case shown="True" "Boolean 9" {
              frame False {
              }
              frame True {
                n3021 = local read "Captured Values 2"() -> (w4267:dbl[][])
                n3022 = Index Array(array=w4267, index (col) #1=0 ("disabled index (col)"), index (col) #2=1 ("index (col)")) -> (element #1=w4270:dbl[], element #2=w4269:dbl[])  [unwired: 2 in]
                n3023 = call <vilib>:"Linear Fit.vi"("Y"=w4270, "X"=w4269) -> ("slope"=→"Slope":dbl, "intercept"=→"Intercept":dbl)  [unwired: 9 in, 3 out]
                n3024 = local write "Boolean 9"(FALSE ("Boolean 9")) -> ()
              }
            }
            n3025 = case shown="True" "Boolean 7" {
              frame False {
              }
              frame True {
                n3026 = local write "Captured Values 2"(dbl[][] [] ("Captured Values")) -> ()
                n3027 = local write "Boolean 7"(FALSE ("Boolean 7")) -> ()
              }
            }
            n3028 = Concatenate Strings("COMMAND 2", "\r", "\n") -> (w4244:string)
            n3029 = case shown="True" "Measure 2" {
              tunnel: w4242 -> [w4277 w4283]
              tunnel: w4241 -> [w4276 w4282]
              tunnel: [w4277 w4281] -> w4240
              tunnel: [w4276 w4280] -> w4239
              tunnel: w4244 -> [_ w4279]
              frame False {
              }
              frame True {
                n3030 = local write "Measure 2"(FALSE ("WRITE")) -> ()
                n3031 = VISA Write(VISA resource name=w4283, write buffer=w4279, error in (no error)=w4282) -> (VISA resource name out=w4281:refnum<visa-resource-name>, error out=w4280:errorcluster)  [unwired: 1 out]
              }
            }
          }
          frame Error {
            w4372 = u16 10 items=["1.0"=10, "1.5"=15, "2.0"=20] ("stop bits (10: 1 bit)")
            n3032 = Wait (ms)(milliseconds to wait=u32 20) -> ()  [unwired: 1 out]
            n3033 = VISA Close(VISA resource name=w4374, error in (no error)=w4380) -> (error out=w4379:errorcluster)
            n3034 = call <vilib>:"Clear Errors.vi"("error in (no error)"=w4379) -> ("error out"=w4378:errorcluster)  [unwired: 5 in, 1 out]
            n3035 = call-poly "VISA Configure Serial Port"("VISA resource name"="Laser Disp Sensor", "timeout (10sec)"=u32 200, "Enable Termination\nChar (T)"=TRUE ("Enable Termination\nChar (T)"), "baud rate (9600)"=u32 921600, "error in (no error)"=w4378, "stop bits (10: 1 bit)"=w4372) -> ("VISA resource name out"=w4382:refnum<visa-resource-name>, "error out"=w4381:errorcluster)  [unwired: 8 in]
          }
        }
        n3036 = local read "EXIT"() -> (w4216:bool)
      }
      n3037 = VISA Close(VISA resource name=w4212, error in (no error)=w4213) -> (error out=w4211:errorcluster)
      n3038 = call <vilib>:"Clear Errors.vi"("error in (no error)"=w4211) -> ()  [unwired: 5 in, 2 out]
    }
  }
  n3039 = case shown="True" "Case Constant\n(See Context Help) 9" {
    tunnel: w16 -> [_ w4383]
    frame False {
    }
    frame True {
      n3040 = while {
        tunnel: [w4394] -> _
        shift-right: [w4391] -> w4385
        shift-left: _ -> [w4393]
        shift-right: [w4392] -> w4386
        shift-left: errorcluster {"status"=TRUE, "code"=0, "source"="Init"} ("error out") -> [w4390]
        tunnel: w4383 -> [_]
        i -> [w4394]
        stop <- w4388 stop-if-true
        n3041 = flat-sequence {
          tunnel: w4390 -> [w4485]
          tunnel: [w4485] -> w4389
          frame #0 {
            n3042 = Wait (ms)(milliseconds to wait=u32 50) -> ()  [unwired: 1 out]
          }
        }
        n3043 = case shown="No Error" w4389 {
          selector: w4389 -> [w4435 w4478]
          tunnel: w4393 -> [w4434 w4477]
          tunnel: [w4401 w4468] -> w4392
          tunnel: [w4402 w4476] -> w4391
          frame No Error {
            w4428 = T17 {"Mode"=enum."RTU", "Slave Address"=1} ("Serial Parameters")
            n3044 = call-poly <vilib>:"MB Serial Master Query (poly).vi"("VISA resource name"=w4434, "Starting Address"=i16 1000, "Quantity"=u16 1, "Timeout"=u32 1000, "error in"=w4435, "Serial Parameters"=w4428) -> ("VISA resource name out"=w4429:refnum<visa-resource-name>, "Input Registers"=w4431:u16[], "error out"=w4427:errorcluster)  [unwired: 10 in, 1 out]
            n3045 = Random Number (0-1)() -> (number: 0 to 1=w4416:dbl)
            n3046 = Index Array(array=w4431, index=0) -> (element=w4426:u16)
            n3047 = Subtract(x=w4416, y=0.5) -> (x-y=w4415:dbl)
            n3048 = Divide(x=w4426, y=10 ("index")) -> (x/y=w4420:dbl)
            n3049 = Multiply(x=w4415, y=0.5) -> (x*y=w4414:dbl)
            n3050 = Add(x=w4420, y=w4414) -> (x+y=w4419:dbl)
            n3051 = local read "Amb temp"() -> (w4403:dbl)
            n3052 = Multiply(x=w4419, y=0.2) -> (x*y=w4423:dbl)
            n3053 = Multiply(x=w4403, y=0.8) -> (x*y=w4421:dbl)
            n3054 = Add(x=w4423, y=w4421) -> (x+y=w4404:dbl)
            n3055 = local read "set temp old"() -> (w4398:dbl)
            n3056 = local write "Amb temp"(w4404) -> ()
            n3057 = Select(t="SetTemp 2", s="Heater", f=100.0) -> (s? t:f=w4399:dbl)
            n3058 = Not Equal?(x=w4399, y=w4398) -> (x != y?=w4397:bool)
            n3059 = case shown="True" w4397 {
              tunnel: w4429 -> [w4463 w4465]
              tunnel: [w4462 w4465] -> w4409
              tunnel: w4427 -> [w4461 w4464]
              tunnel: [w4460 w4464] -> w4407
              tunnel: w4399 -> [w4455 _]
              tunnel: w4428 -> [w4457 w4466]
              tunnel: [w4457 w4466] -> w4410
              frame True {
                n3060 = Multiply(x=w4455, y=10 ("index")) -> (x*y=w4454:dbl)
                n3061 = call-poly <vilib>:"MB Serial Master Query (poly).vi"("VISA resource name"=w4463, "Address"=u16 0, "Holding Register"=w4454, "Timeout"=u32 1000, "error in"=w4461, "Serial Parameters"=w4457) -> ("VISA resource name out"=w4462:refnum<visa-resource-name>, "error out"=w4460:errorcluster)  [unwired: 11 in, 1 out]
                "set temp old" <- w4455
              }
              frame False {
              }
            }
            n3062 = flat-sequence {
              tunnel: [w4436] -> _
              tunnel: [w4436] -> w4406
              tunnel: w4407 -> [w4436]
              frame #0 {
                n3063 = Wait (ms)(milliseconds to wait=u32 100) -> ()  [unwired: 1 out]
              }
            }
            n3064 = call "Elapsed Time12"("Time Target (s)"=2.0, "Auto Reset"=TRUE) -> ("Time has Elapsed"=w4411:bool)  [unwired: 10 in, 7 out]
            n3065 = case shown="True" w4411 {
              tunnel: w4410 -> [w4440 w4453]
              tunnel: [w4440 w4453] -> _
              tunnel: [w4439 w4451] -> w4402
              tunnel: w4409 -> [w4439 w4452]
              tunnel: [w4438 w4449] -> w4401
              tunnel: w4406 -> [w4438 w4450]
              frame False {
              }
              frame True {
                n3066 = call-poly <vilib>:"MB Serial Master Query (poly).vi"("VISA resource name"=w4452, "Starting Address"=i16 1003 ("Addr"), "Quantity"=u16 1, "Timeout"=u32 1000, "error in"=w4450, "Serial Parameters"=w4453) -> ("VISA resource name out"=w4451:refnum<visa-resource-name>, "Input Registers"=w4446:u16[], "error out"=w4449:errorcluster)  [unwired: 10 in, 1 out]
                n3067 = Index Array(array=w4446, index=0) -> (element=w4445:u16)
                n3068 = Divide(x=w4445, y=u16 10) -> (x/y=w4441:dbl)
                n3069 = local write "set temp old"(w4441) -> ()
                n3070 = local write "SetTemp"(w4441) -> ()
              }
            }
            "Error Code" <- w4401
            n3071 = Unbundle(w4401) -> ("status"=→"TK4 status":bool)  [unwired: 2 out]
            "SetTemp" <- "SetTemp 2"
          }
          frame Error {
            w4480 = u16 0 items=["None", "Odd", "Even", "Mark", "Space"] ("Parity")
            w4481 = u16 0 items=["None", "XON/XOFF", "RTS/CTS", "XON/XOFF & RTS/CTS", "DTR/DSR", "XON/XOFF & DTR/DSR"] ("Flow Control")
            n3072 = VISA Clear(VISA resource name=w4477, error in (no error)=w4478) -> (VISA resource name out=w4471:refnum<visa-resource-name>, error out=w4469:errorcluster)
            n3073 = VISA Close(VISA resource name=w4471, error in (no error)=w4469) -> (error out=w4470:errorcluster)
            n3074 = call <vilib>:"Clear Errors.vi"("error in (no error)"=w4470) -> ("error out"=w4479:errorcluster)  [unwired: 5 in, 1 out]
            n3075 = Unbundle By Name(T17 {"Mode"=enum."RTU", "Slave Address"=1} ("input cluster")) -> ("Mode"=w4482:enum16{"RTU", "ASCII"})
            n3076 = call <vilib>:"MB Serial Init.vi"("Timeout"=u32 100, "Flow Control"=w4481, "Mode"=w4482, "error in (no error)"=w4479, "Parity"=w4480, "Baud Rate"=u32 9600, "VISA resource name"="Lubrication System COM Port :") -> ("error out"=w4468:errorcluster, "VISA resource name out"=w4476:refnum<visa-resource-name>)  [unwired: 3 in]
            n3077 = local write "set temp old"(0.0 ("set temp old")) -> ()
            n3078 = Unbundle(w4468) -> ("status"=w4467:bool)  [unwired: 2 out]
            n3079 = case shown="True" w4467 {
              selector: w4467 -> [_ w4484]
              frame False {
              }
              frame True {
                n3080 = local write "TK4 status"(w4484) -> ()
              }
            }
          }
        }
        n3081 = local read "EXIT"() -> (w4388:bool)
      }
      n3082 = VISA Close(VISA resource name=w4385, error in (no error)=w4386) -> (error out=w4384:errorcluster)
      n3083 = call <vilib>:"Clear Errors.vi"("error in (no error)"=w4384) -> ()  [unwired: 5 in, 2 out]
    }
  }
  "file count" <- 0 ("file count")
